vi "Main FP.vi"() -> ()   [LabVIEW 2017]
doc: "Custom software for Stepper dyno control to monitor the torque and RPM while changing the torque of the dyno. Note that the drive in the dyno should be set to torque mode. LabVIEW doesn't have a capability to determine if the dyno is in torque mode."
uses:
  DAQ States.ctl
panel:
  in  "Duration":dbl=5.0 caption="Sample Duration"
  in  "Tab Control":enum32{"Constant", "Square"}(tab)
  in  "Current Settings":T1 {"Torque Percentage" min=0 max=100 format="%#_6f"}
  in  "Update Square":bool
  in  "Sq Wave Properties":T2 {"Duty Cycle(%)" min=0 max=100}
  out "Average Input":dbl[](array[numeric])
  in  "AI List":i32[](listbox)
  in  "Pause":bool
  in  "Save RPM":bool
  in  "Save AI":bool
  out "Average RPM":dbl
  out "AI Graph":waveform(dbl)[](graph)
  out "RPM Graph":cluster{"X":dbl, "Y":dbl}[](graph)
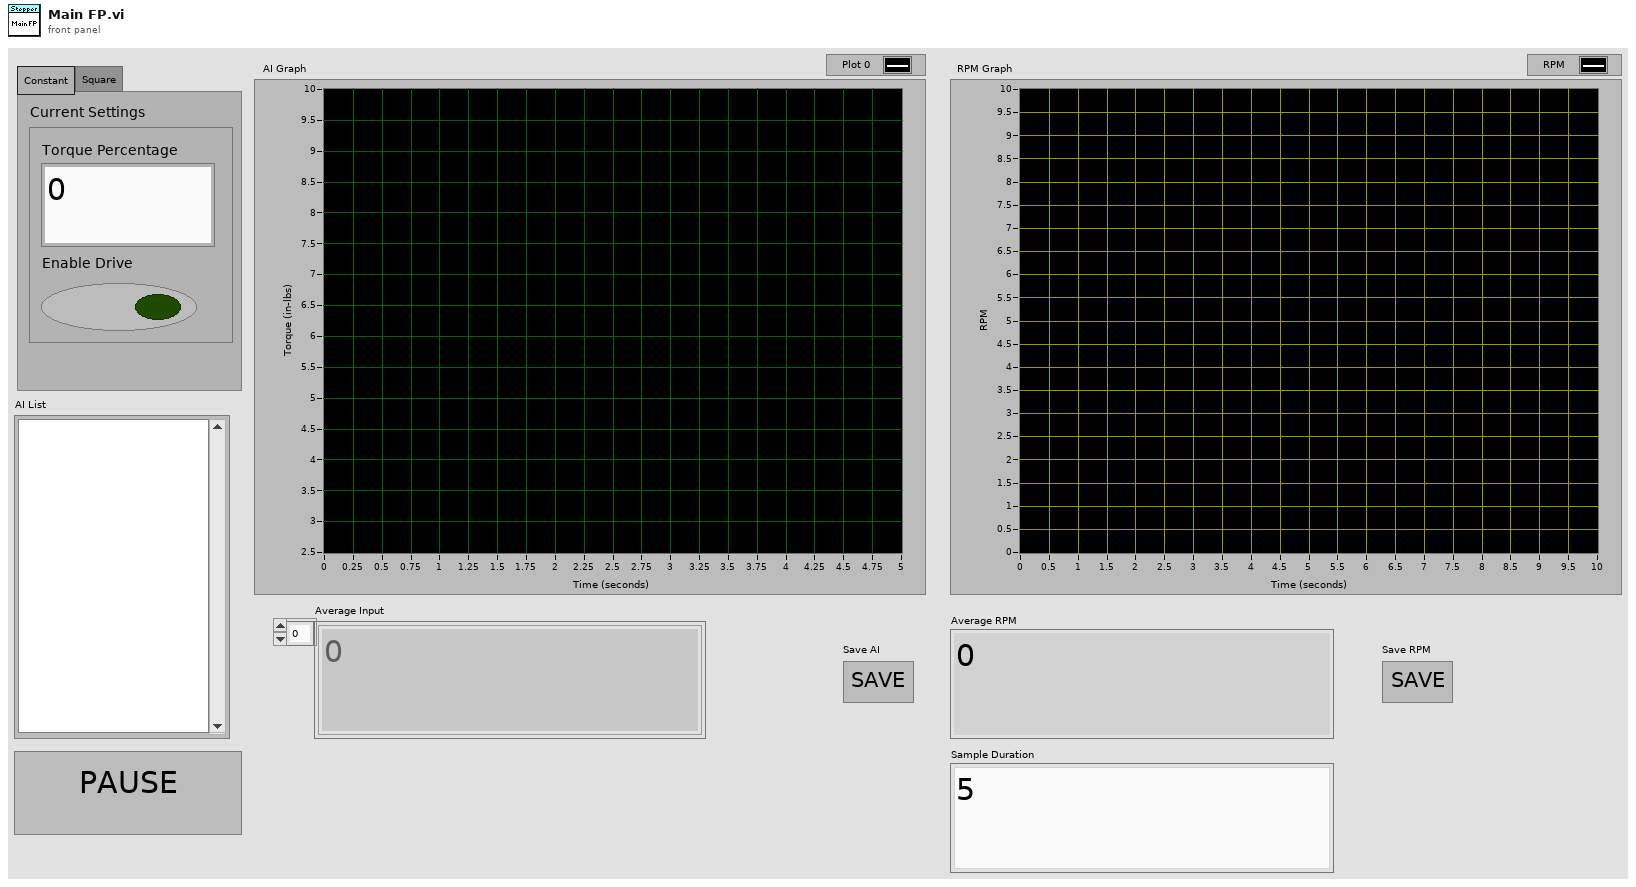
[diagram p1: front panel]
types:
  T1 = cluster{"Torque Percentage":sgl, "Enable Drive":bool}
  T2 = cluster{"Minimum":sgl, "Maximum":sgl, "Duty Cycle(%)":sgl, "Frequency(Hz))":sgl}
  T3 = cluster{"AI Graph":refnum<vi>, "RPM Graph":refnum<vi>, "Average Input":refnum<vi>, "Average RPM":refnum<vi>, "AI List":refnum<vi>}
  T4 = typedef "DAQ States.ctl" = enum16{"Init", "Exit", "Update Settings", "Pause", "Update Square", "Update Duration"}
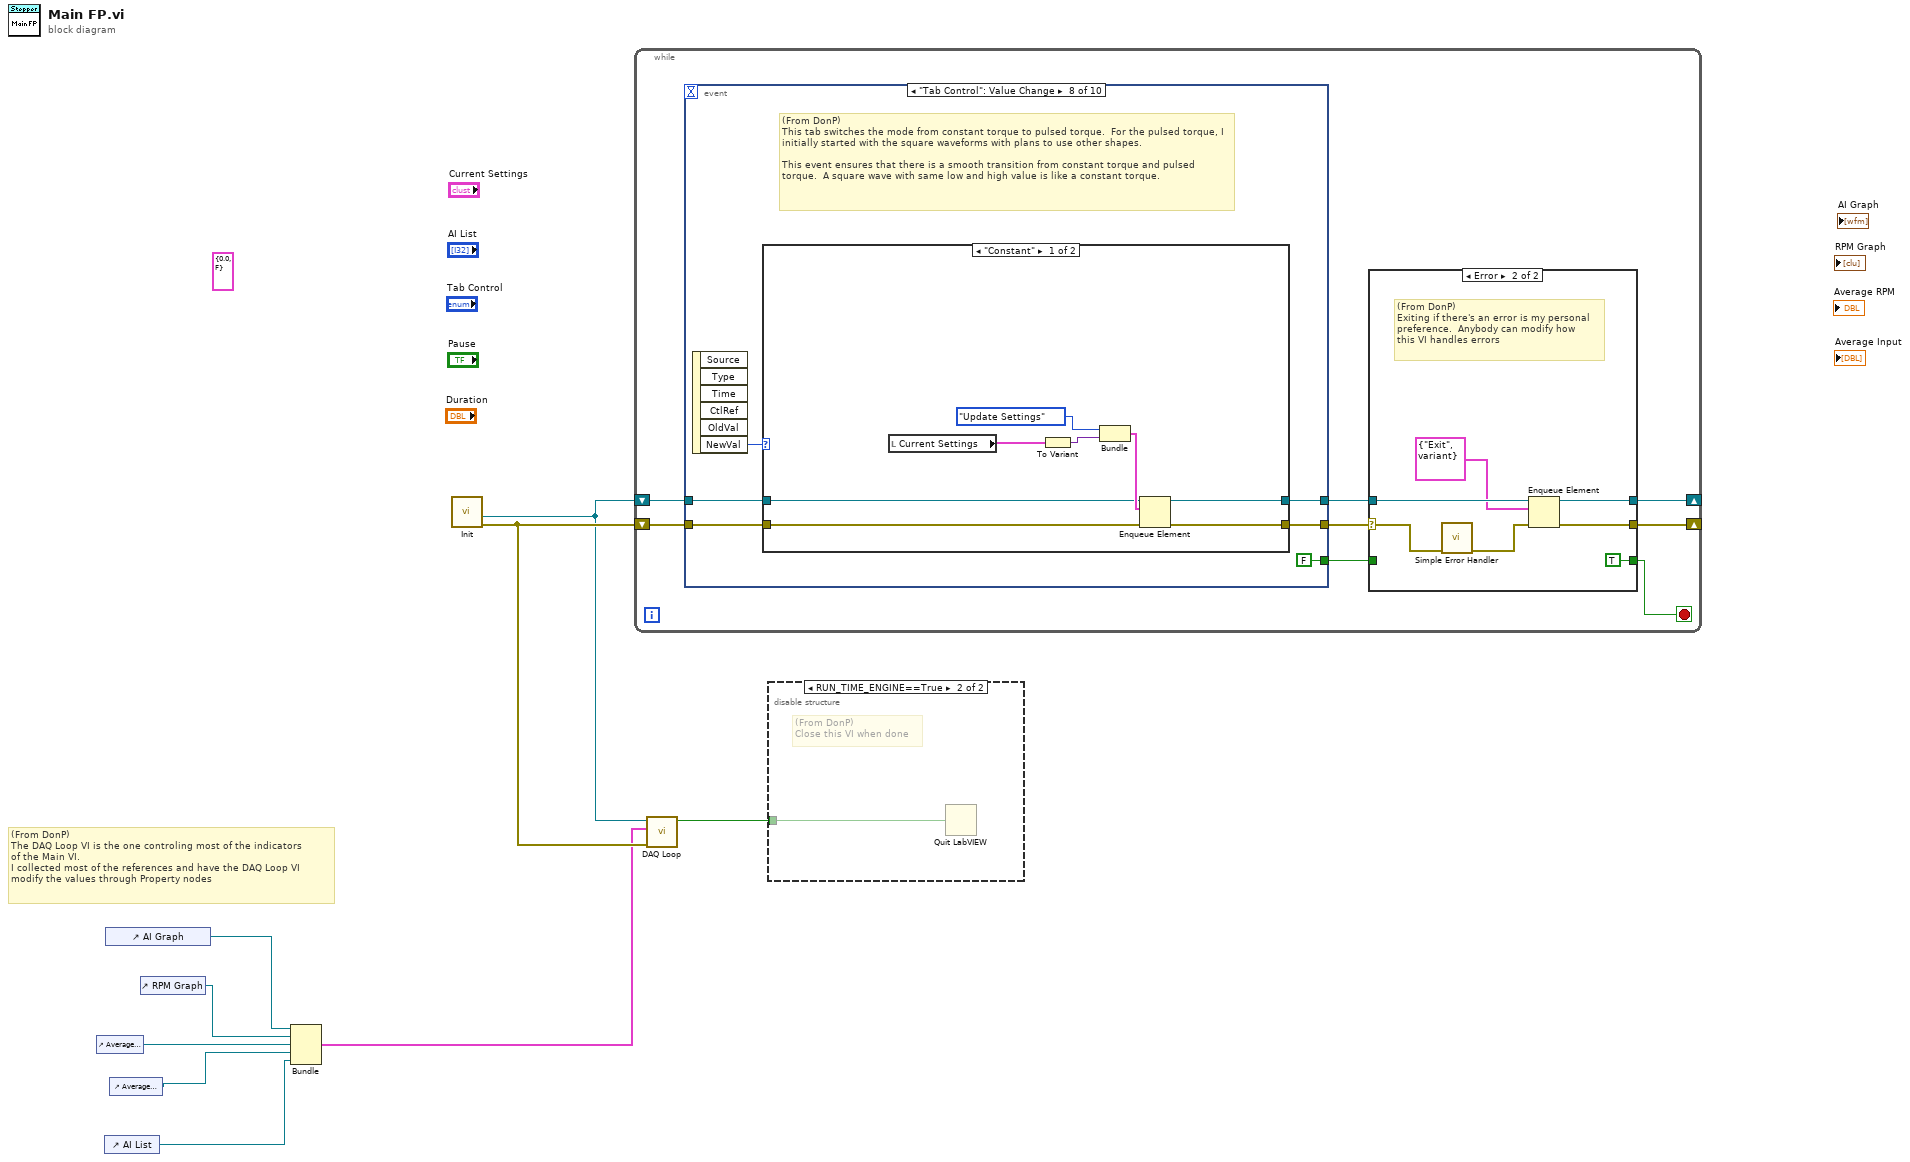
[diagram p0: block diagram]
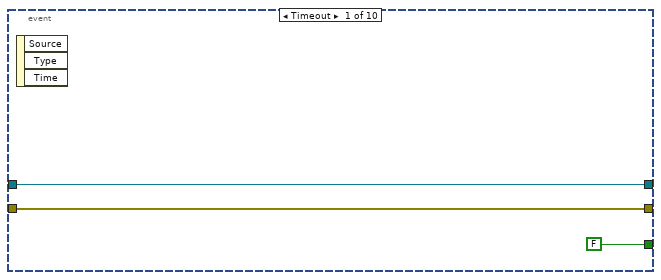
[diagram p4: hidden frame]
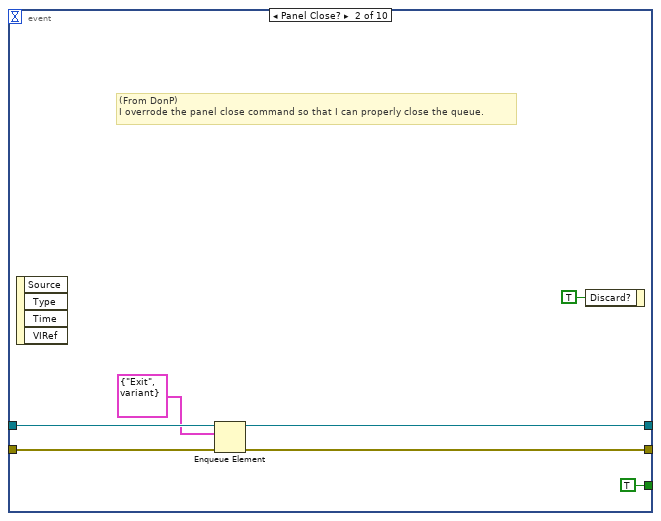
[diagram p5: hidden frame]
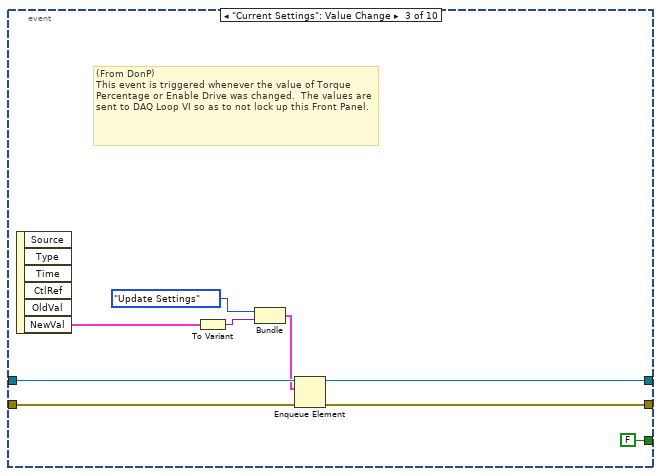
[diagram p6: hidden frame]
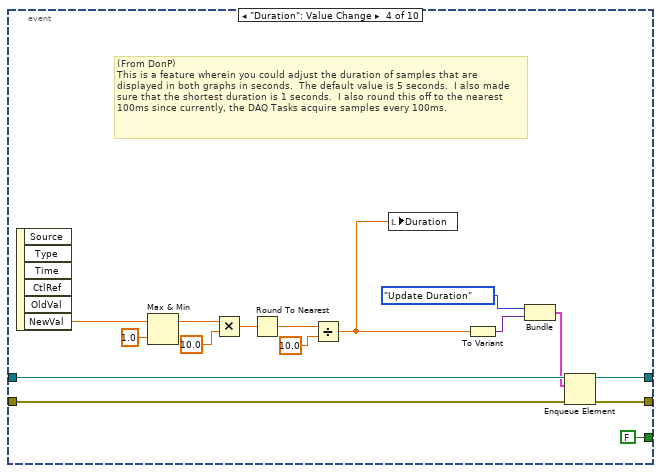
[diagram p7: hidden frame]
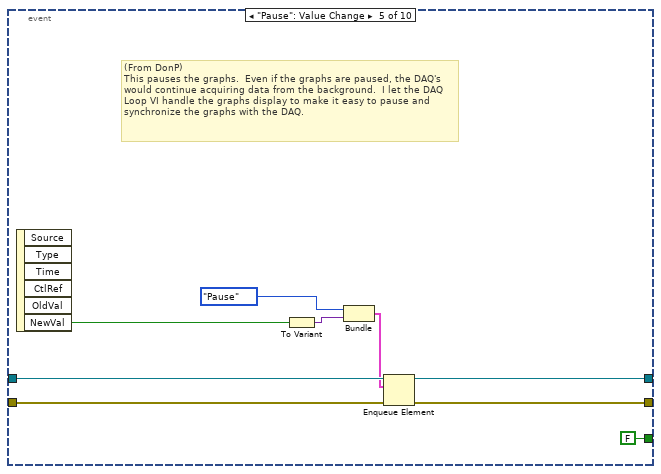
[diagram p8: hidden frame]
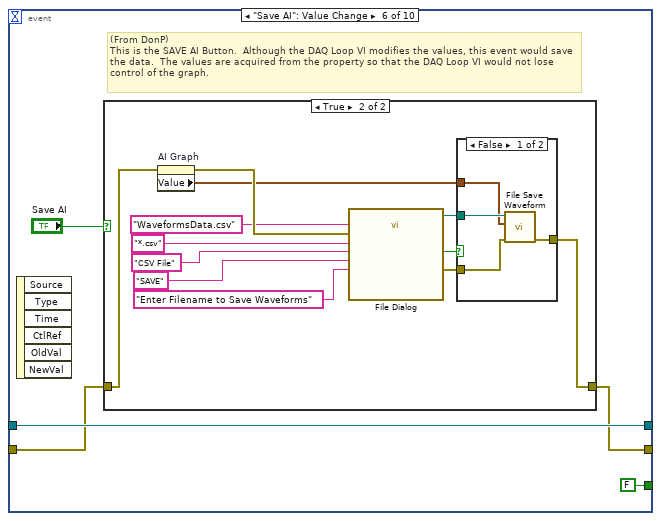
[diagram p9: hidden frame]
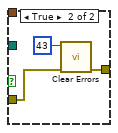
[diagram p11: hidden frame]
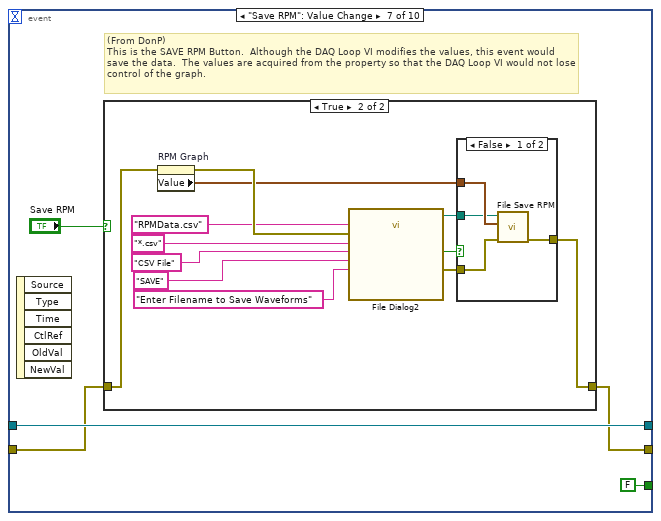
[diagram p12: hidden frame]
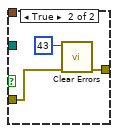
[diagram p14: hidden frame]
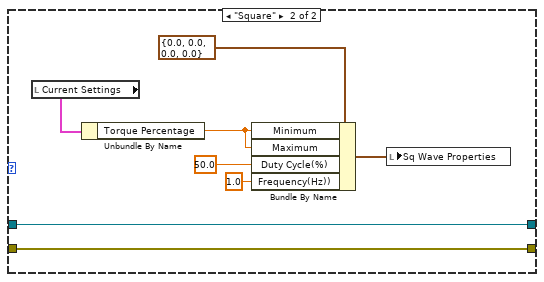
[diagram p15: hidden frame]
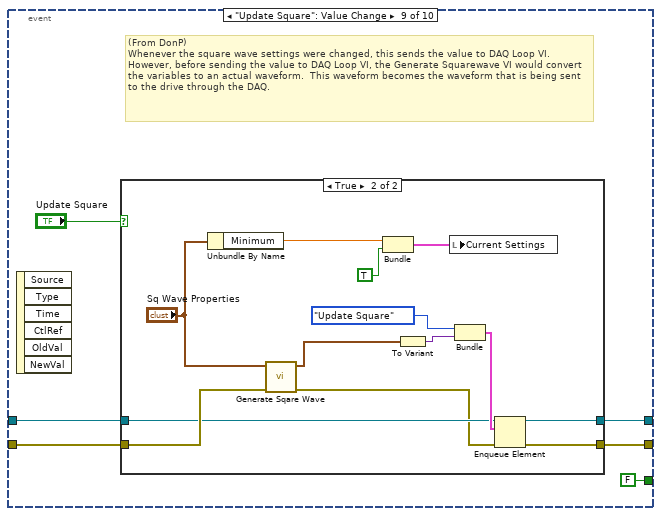
[diagram p16: hidden frame]
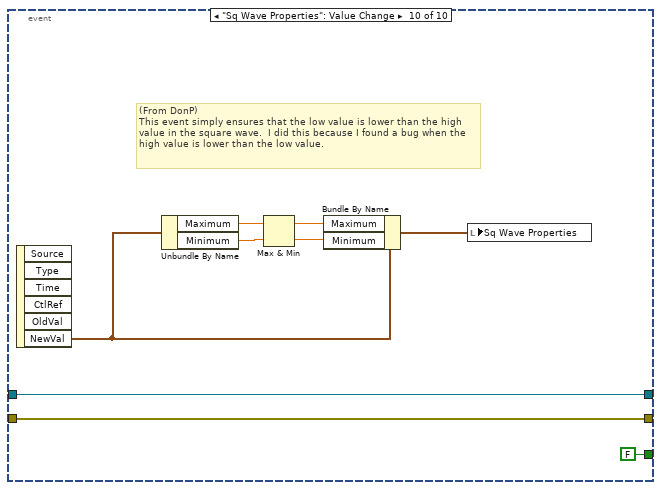
[diagram p18: hidden frame]
diagram:
  (unwired) T1 {"Torque Percentage"=0.0, "Enable Drive"=FALSE} ("Current Settings")
  # "(From DonP)\nThe DAQ Loop VI is the one controling most of the indicators\nof the Main VI.\nI collected most of the references and have the DAQ Loop VI\nmodify the values through Property nodes"
  n1 = control-ref of="Average Input"() -> (w1:refnum<vi>)
  n2 = control-ref of="AI List"() -> (w2:refnum<vi>)
  n3 = control-ref of="AI Graph"() -> (w6:refnum<vi>)
  n4 = control-ref of="Average RPM"() -> (w3:refnum<vi>)
  n5 = control-ref of="RPM Graph"() -> (w5:refnum<vi>)
  n6 = Bundle("AI Graph"=w6, "RPM Graph"=w5, "Average Input"=w1, "Average RPM"=w3, "AI List"=w2) -> (w4:T3)  [unwired: 1 in]
  n7 = call "Init.vi"() -> ("error out"=w9:errorcluster, "DAQ Queue"=w8:refnum<queue>)  [unwired: 10 in]
  n8 = while {
    shift-right: [w12] -> _
    shift-left: w9 -> [w16]
    shift-right: [w11] -> _
    shift-left: w8 -> [w17]
    stop <- w13 stop-if-true
    n9 = event shown="[7] \"Tab Control\": Value Change" {
      selector: _ -> [_ _ _ _ _ _ _ _ _ _]
      dyn-events: _ -> [_ _ _ _ _ _ _ _ _ _]
      timeout: _ -> [_ _ _ _ _ _ _ _ _ _]
      tunnel: w17 -> [w30 w36 w45 w62 w70 w75 w100 w125 w148 w167]
      tunnel: w16 -> [w29 w35 w44 w61 w69 w74 w99 w124 w147 w166]
      tunnel: [w30 w33 w40 w57 w65 w75 w100 w122 w146 w167] -> w10
      tunnel: [w29 w32 w39 w56 w64 w73 w98 w123 w145 w166] -> w15
      tunnel: [FALSE TRUE FALSE FALSE FALSE FALSE FALSE FALSE FALSE FALSE] -> w14
      event Timeout {
        n10 = event-data() -> ()  [unwired: 1 in, 3 out]
      }
      event Panel Close? {
        # "(From DonP)\nI overrode the panel close command so that I can properly close the queue."
        n11 = event-data() -> ()  [unwired: 1 in, 4 out]
        n12 = Enqueue Element(queue=w36, element=cluster{"State":T4, "Data":variant} {"State"=enum."Exit", "Data"=variant}, error in (no error)=w35) -> (queue out=w33:refnum<queue>, error out=w32:errorcluster)  [unwired: 1 in, 1 out]
        n13 = event-data("Discard?"=TRUE) -> ()  [unwired: 1 in, 1 out]
      }
      event "Current Settings": Value Change {
        # "(From DonP)\nThis event is triggered whenever the value of Torque Percentage or Enable Drive was changed.  The values are sent to DAQ Loop VI so as to not lock up this Front Panel."
        n14 = event-data() -> ("NewVal"=w46:T1)  [unwired: 1 in, 5 out]
        n15 = To Variant(anything=w46) -> (Variant=w43:variant)
        n16 = Bundle("DAQ States"=DAQ_States."Update Settings", "Variant"=w43) -> (w41:cluster{"DAQ States":T4, "Variant":variant})  [unwired: 1 in]
        n17 = Enqueue Element(queue=w45, element=w41, error in (no error)=w44) -> (queue out=w40:refnum<queue>, error out=w39:errorcluster)  [unwired: 1 in, 1 out]
      }
      event "Duration": Value Change {
        # "(From DonP)\nThis is a feature wherein you could adjust the duration of samples that are displayed in both graphs in seconds.  The default value is 5 seconds.  I also made sure that the shortest duration is 1 seconds.  I also round this off to the nearest 100ms since currently, the DAQ Tasks acquire samples every 100ms."
        n18 = event-data() -> ("NewVal"=w54:dbl)  [unwired: 1 in, 5 out]
        n19 = Max & Min(x=w54, y=1.0) -> (max(x,y)=w52:dbl)  [unwired: 1 out]
        n20 = Multiply(x=w52, y=10.0) -> (x*y=w50:dbl)
        n21 = Round To Nearest(number=w50) -> (nearest integer value=w49:dbl)
        n22 = Divide(x=w49, y=10.0) -> (x/y=w47:dbl)
        n23 = local write "Duration"(w47) -> ()
        n24 = To Variant(anything=w47) -> (Variant=w60:variant)
        n25 = Bundle("DAQ States"=DAQ_States."Update Duration", "Variant"=w60) -> (w58:cluster{"DAQ States":T4, "Variant":variant})  [unwired: 1 in]
        n26 = Enqueue Element(queue=w62, element=w58, error in (no error)=w61) -> (queue out=w57:refnum<queue>, error out=w56:errorcluster)  [unwired: 1 in, 1 out]
      }
      event "Pause": Value Change {
        # "(From DonP)\nThis pauses the graphs.  Even if the graphs are paused, the DAQ's would continue acquiring data from the background.  I let the DAQ Loop VI handle the graphs display to make it easy to pause and synchronize the graphs with the DAQ."
        n27 = event-data() -> ("NewVal"=w71:bool)  [unwired: 1 in, 5 out]
        n28 = To Variant(anything=w71) -> (Variant=w68:variant)
        n29 = Bundle("DAQ States"=DAQ_States."Pause", "Variant"=w68) -> (w66:cluster{"DAQ States":T4, "Variant":variant})  [unwired: 1 in]
        n30 = Enqueue Element(queue=w70, element=w66, error in (no error)=w69) -> (queue out=w65:refnum<queue>, error out=w64:errorcluster)  [unwired: 1 in, 1 out]
      }
      event "Save AI": Value Change {
        # "(From DonP)\nThis is the SAVE AI Button.  Although the DAQ Loop VI modifies the values, this event would save the data.  The values are acquired from the property so that the DAQ Loop VI would not lose control of the graph."
        n31 = event-data() -> ()  [unwired: 1 in, 6 out]
        n32 = case shown="True" "Save AI" {
          tunnel: w74 -> [w77 w89]
          tunnel: [w77 w84] -> w73
          frame False {
          }
          frame True {
            n33 = property on="AI Graph" class="WFGraph (strict)"(error in=w89) -> (error out=w88:errorcluster, "Value"=w86:waveform(dbl)[])  [unwired: 1 in, 1 out]
            n34 = call "File Dialog"("prompt"="Enter Filename to Save Waveforms", "button label"="SAVE", "default name"="WaveformsData.csv", "error in"=w88, "pattern (all files)"="*.csv", "pattern label"="CSV File") -> ("selected path"=w87:path, "cancelled"=w78:bool, "error out"=w85:errorcluster)  [unwired: 6 in, 1 out]
            n35 = case shown="False" w78 {
              tunnel: w87 -> [w93 _]
              tunnel: w86 -> [w92 _]
              tunnel: w85 -> [w91 w95]
              tunnel: [w90 w96] -> w84
              frame False {
                n36 = call "File Save Waveform.vi"("error in (no error)"=w91, "Waveforms"=w92, "File Path"=w93) -> ("error out"=w90:errorcluster)  [unwired: 8 in]
              }
              frame True {
                n37 = call <vilib>:"Clear Errors.vi"("error in (no error)"=w95, "specific error code to clear (0: all)"=43) -> ("error out"=w96:errorcluster)  [unwired: 4 in, 1 out]
              }
            }
          }
        }
      }
      event "Save RPM": Value Change {
        # "(From DonP)\nThis is the SAVE RPM Button.  Although the DAQ Loop VI modifies the values, this event would save the data.  The values are acquired from the property so that the DAQ Loop VI would not lose control of the graph."
        n38 = event-data() -> ()  [unwired: 1 in, 6 out]
        n39 = case shown="True" "Save RPM" {
          tunnel: w99 -> [w102 w114]
          tunnel: [w102 w109] -> w98
          frame False {
          }
          frame True {
            n40 = property on="RPM Graph" class="XYGraph (strict)"(error in=w114) -> (error out=w113:errorcluster, "Value"=w111:cluster{"X":dbl, "Y":dbl}[])  [unwired: 1 in, 1 out]
            n41 = call "File Dialog2"("prompt"="Enter Filename to Save Waveforms", "button label"="SAVE", "default name"="RPMData.csv", "error in"=w113, "pattern (all files)"="*.csv", "pattern label"="CSV File") -> ("selected path"=w112:path, "cancelled"=w103:bool, "error out"=w110:errorcluster)  [unwired: 6 in, 1 out]
            n42 = case shown="False" w103 {
              tunnel: w112 -> [w115 _]
              tunnel: w111 -> [w116 _]
              tunnel: w110 -> [w117 w120]
              tunnel: [w118 w121] -> w109
              frame False {
                n43 = call "File Save RPM.vi"("error in (no error)"=w117, "XY Graph"=w116, "File Name"=w115) -> ("error out"=w118:errorcluster)  [unwired: 8 in]
              }
              frame True {
                n44 = call <vilib>:"Clear Errors.vi"("error in (no error)"=w120, "specific error code to clear (0: all)"=43) -> ("error out"=w121:errorcluster)  [unwired: 4 in, 1 out]
              }
            }
          }
        }
      }
      event "Tab Control": Value Change {
        # "(From DonP)\nThis tab switches the mode from constant torque to pulsed torque.  For the pulsed torque, I initially started with the square waveforms with plans to use other shapes.\n\nThis event ensures that there is a smooth transition from constant torque and pulsed torque.  A square wave with same low and high value is like a constant torque."
        n45 = event-data() -> ("NewVal"=w126:enum32{"Constant", "Square"})  [unwired: 1 in, 5 out]
        n46 = case shown="\"Constant\"" w126 {
          tunnel: w125 -> [w132 w143]
          tunnel: w124 -> [w131 w142]
          tunnel: [w130 w142] -> w123
          tunnel: [w129 w143] -> w122
          frame "Constant" {
            n47 = local read "Current Settings"() -> (w128:T1)
            n48 = To Variant(anything=w128) -> (Variant=w135:variant)
            n49 = Bundle("DAQ States"=DAQ_States."Update Settings", "Variant"=w135) -> (w134:cluster{"DAQ States":T4, "Variant":variant})  [unwired: 1 in]
            n50 = Enqueue Element(queue=w132, element=w134, error in (no error)=w131) -> (queue out=w129:refnum<queue>, error out=w130:errorcluster)  [unwired: 1 in, 1 out]
          }
          frame "Square" {
            n51 = local read "Current Settings"() -> (w141:T1)
            n52 = Unbundle By Name(w141) -> ("Torque Percentage"=w138:sgl)
            n53 = Bundle By Name(cluster=T2 {"Minimum"=0.0, "Maximum"=0.0, "Duty Cycle(%)"=0.0, "Frequency(Hz))"=0.0} ("Sq Wave Properties"), "Minimum"=w138, "Maximum"=w138, "Duty Cycle(%)"=sgl 50.0, "Frequency(Hz))"=sgl 1.0) -> (w139:T2)
            n54 = local write "Sq Wave Properties"(w139) -> ()
          }
        }
      }
      event "Update Square": Value Change {
        # "(From DonP)\nWhenever the square wave settings were changed, this sends the value to DAQ Loop VI.  However, before sending the value to DAQ Loop VI, the Generate Squarewave VI would convert the variables to an actual waveform.  This waveform becomes the waveform that is being sent to the drive through the DAQ."
        n55 = event-data() -> ()  [unwired: 1 in, 6 out]
        n56 = case shown="True" "Update Square" {
          tunnel: w148 -> [w151 w158]
          tunnel: w147 -> [w150 w159]
          tunnel: [w151 w161] -> w146
          tunnel: [w150 w160] -> w145
          frame False {
          }
          frame True {
            n57 = Unbundle By Name("Sq Wave Properties") -> ("Minimum"=w154:sgl)
            n58 = call "Generate Sqare Wave.vi"("error in (no error)"=w159, "Sq Wave Properties"="Sq Wave Properties") -> ("error out"=w157:errorcluster, "Waveform"=w156:waveform(dbl))  [unwired: 8 in]
            n59 = Bundle("Minimum"=w154, TRUE) -> (w152:cluster{"Minimum":sgl, bool})  [unwired: 1 in]
            n60 = To Variant(anything=w156) -> (Variant=w164:variant)
            n61 = local write "Current Settings"(w152) -> ()
            n62 = Bundle("DAQ States"=DAQ_States."Update Square", "Variant"=w164) -> (w162:cluster{"DAQ States":T4, "Variant":variant})  [unwired: 1 in]
            n63 = Enqueue Element(queue=w158, element=w162, error in (no error)=w157) -> (queue out=w161:refnum<queue>, error out=w160:errorcluster)  [unwired: 1 in, 1 out]
          }
        }
      }
      event "Sq Wave Properties": Value Change {
        # "(From DonP)\nThis event simply ensures that the low value is lower than the high value in the square wave.  I did this because I found a bug when the high value is lower than the low value."
        n64 = event-data() -> ("NewVal"=w171:T2)  [unwired: 1 in, 5 out]
        n65 = Unbundle By Name(w171) -> ("Maximum"=w173:sgl, "Minimum"=w172:sgl)
        n66 = Max & Min(x=w173, y=w172) -> (max(x,y)=w169:sgl, min(x,y)=w168:sgl)
        n67 = Bundle By Name(cluster=w171, "Maximum"=w169, "Minimum"=w168) -> (w170:T2)
        n68 = local write "Sq Wave Properties"(w170) -> ()
      }
    }
    n69 = case shown="Error" w15 {
      selector: w15 -> [w19 w27]
      tunnel: w14 -> [w20 _]
      tunnel: [w20 TRUE] -> w13
      tunnel: [w19 w25] -> w12
      tunnel: [w18 w23] -> w11
      tunnel: w10 -> [w18 w24]
      frame No Error {
      }
      frame Error {
        # "(From DonP)\nExiting if there's an error is my personal\npreference.  Anybody can modify how\nthis VI handles errors"
        n70 = call <vilib>:"Simple Error Handler.vi"("error in (no error)"=w27) -> ("error out"=w26:errorcluster)  [unwired: 4 in, 4 out]
        n71 = Enqueue Element(queue=w24, element=cluster{"State":T4, "Data":variant} {"State"=enum."Exit", "Data"=variant}, error in (no error)=w26) -> (queue out=w23:refnum<queue>, error out=w25:errorcluster)  [unwired: 1 in, 1 out]
      }
    }
  }
  n72 = call "DAQ Loop.vi"("error in (no error)"=w9, "Reference Cluster"=w4, "DAQ Queue"=w8) -> ("Stop"=w7:bool)  [unwired: 7 in, 1 out]
  n73 = disable-structure shown="RUN_TIME_ENGINE==True" {
    disable-tunnel: w7 -> [_ w174]
    frame condition #0 (active) {
    }
    frame condition #1 {
      # "(From DonP)\nClose this VI when done"
      n74 = Quit LabVIEW(quit? (T)=w174) -> ()
    }
  }
